vi "Zoom_Faktor.vi"(9 "Limit to 1x":bool, 10 "Array":bool[](array[boolean]), 11 "ZoomInteger 2":cluster{"X":i32, "Y":i32}) -> (2 "X":dbl, 3 "ZoomInteger":cluster{"X":i32, "Y":i32})   [LabVIEW 2011]
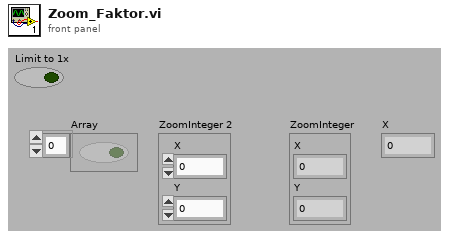
[diagram p1: front panel]
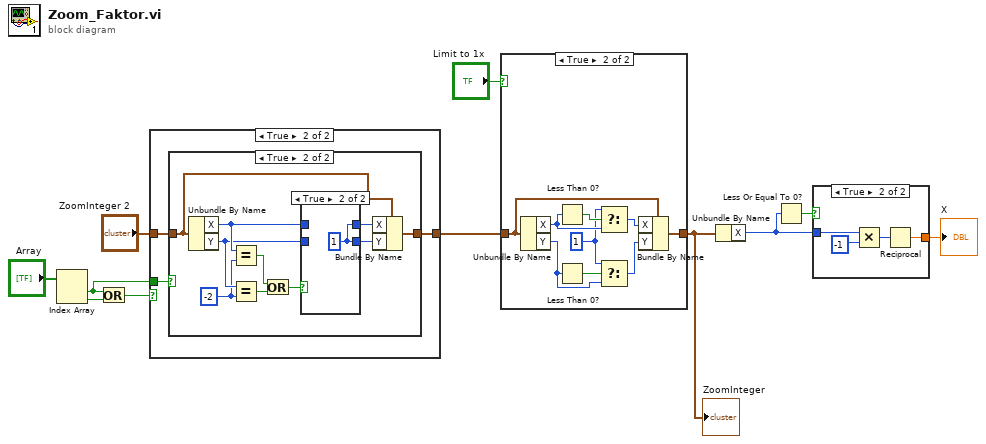
[diagram p0: block diagram]
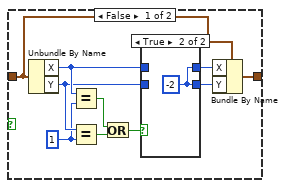
[diagram p5: hidden frame]
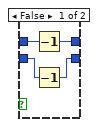
[diagram p6: hidden frame]
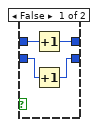
[diagram p7: hidden frame]
diagram:
  n1 = Index Array(array="Array") -> (element #1=w11:bool, element #2=w10:bool)  [unwired: 2 in]
  n2 = Or(x=w11, y=w10) -> (x .or. y?=w4:bool)
  n3 = case shown="True" w4 {
    tunnel: w11 -> [_ w15]
    tunnel: "ZoomInteger 2" -> [w12 w14]
    tunnel: [w12 w13] -> w3
    frame False {
    }
    frame True {
      n4 = case shown="True" w15 {
        tunnel: w14 -> [w17 w37]
        tunnel: [w16 w38] -> w13
        frame False {
          w21 = 1 ("y")
          n5 = Unbundle By Name(w17) -> ("X"=w23:i32, "Y"=w22:i32)
          n6 = Equal?(x=w23, y=w21) -> (x = y?=w20:bool)
          n7 = Equal?(x=w22, y=w21) -> (x = y?=w19:bool)
          n8 = Or(x=w20, y=w19) -> (x .or. y?=w18:bool)
          n9 = case shown="True" w18 {
            tunnel: [w29 w30] -> w25
            tunnel: [w28 w30] -> w24
            tunnel: w23 -> [w27 _]
            tunnel: w22 -> [w26 _]
            frame False {
              n10 = Decrement(x=w27) -> (x-1=w29:i32)
              n11 = Decrement(x=w26) -> (x-1=w28:i32)
            }
            frame True {
              w30 = -2
            }
          }
          n12 = Bundle By Name(cluster=w17, "X"=w25, "Y"=w24) -> (w16:cluster{"X":i32, "Y":i32})
        }
        frame True {
          w34 = -2 ("y")
          n13 = Unbundle By Name(w37) -> ("X"=w36:i32, "Y"=w35:i32)
          n14 = Equal?(x=w36, y=w34) -> (x = y?=w33:bool)
          n15 = Equal?(x=w35, y=w34) -> (x = y?=w32:bool)
          n16 = Or(x=w33, y=w32) -> (x .or. y?=w31:bool)
          n17 = case shown="True" w31 {
            tunnel: [w44 w45] -> w40
            tunnel: [w43 w45] -> w39
            tunnel: w36 -> [w42 _]
            tunnel: w35 -> [w41 _]
            frame False {
              n18 = Increment(x=w42) -> (x+1=w44:i32)
              n19 = Increment(x=w41) -> (x+1=w43:i32)
            }
            frame True {
              w45 = 1
            }
          }
          n20 = Bundle By Name(cluster=w37, "X"=w40, "Y"=w39) -> (w38:cluster{"X":i32, "Y":i32})
        }
      }
    }
  }
  n21 = case shown="True" "Limit to 1x" {
    tunnel: w3 -> [w46 w49]
    tunnel: [w46 w48] -> w1
    frame False {
    }
    frame True {
      w47 = 1 ("t")
      n22 = Unbundle By Name(w49) -> ("X"=w54:i32, "Y"=w52:i32)
      n23 = Less Than 0?(x=w54) -> (x < 0?=w55:bool)
      n24 = Less Than 0?(x=w52) -> (x < 0?=w53:bool)
      n25 = Select(t=w47, s=w55, f=w54) -> (s? t:f=w51:i32)
      n26 = Select(t=w47, s=w53, f=w52) -> (s? t:f=w50:i32)
      n27 = Bundle By Name(cluster=w49, "X"=w51, "Y"=w50) -> (w48:cluster{"X":i32, "Y":i32})
    }
  }
  "ZoomInteger" <- w1
  n28 = Unbundle By Name(w1) -> ("X"=w7:i32)
  n29 = Less Or Equal To 0?(x=w7) -> (x <= 0?=w8:bool)
  n30 = case shown="True" w8 {
    tunnel: w7 -> [w56 w60]
    tunnel: [w56 w57] -> w6
    frame False {
    }
    frame True {
      n31 = Multiply(x=w60, y=-1) -> (x*y=w58:i32)
      n32 = Reciprocal(x=w58) -> (1/x=w57:dbl)
    }
  }
  "X" <- w6
